vi "read_csv.vi"(7 "Read":bool, 11 "Read File:":path) -> (1 "Header":string[][](array[string]), 2 "# Header Lines":i32, 3 "File Data":T1)   [LabVIEW 2019]
uses:
  <vilib>/Analysis/Matrix/Datatypes/RealMatrix.ctl
  <vilib>/Utility/file.llb/Read Delimited Spreadsheet (DBL).vi
  <vilib>/Utility/file.llb/Read Delimited Spreadsheet (string).vi
  <vilib>/Analysis/Matrix/Numeric/Conversions/Array To Matrix - RA2.vi
  <vilib>/Analysis/Matrix/NI_Matrix.lvlib
panel:
  out "Head Row?":bool
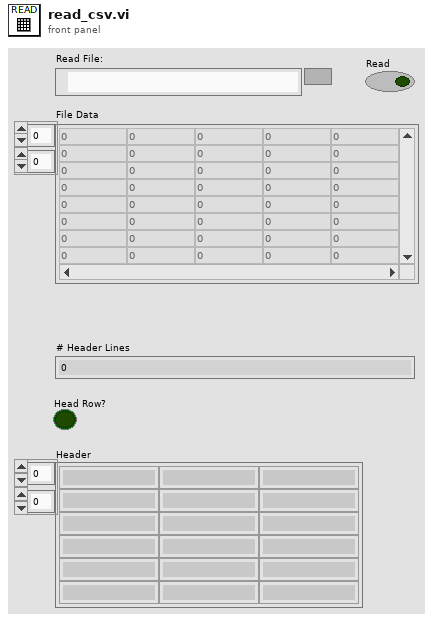
[diagram p1: front panel]
types:
  T1 = typedef "NI_Matrix.lvlib/RealMatrix.ctl" = dbl[][]
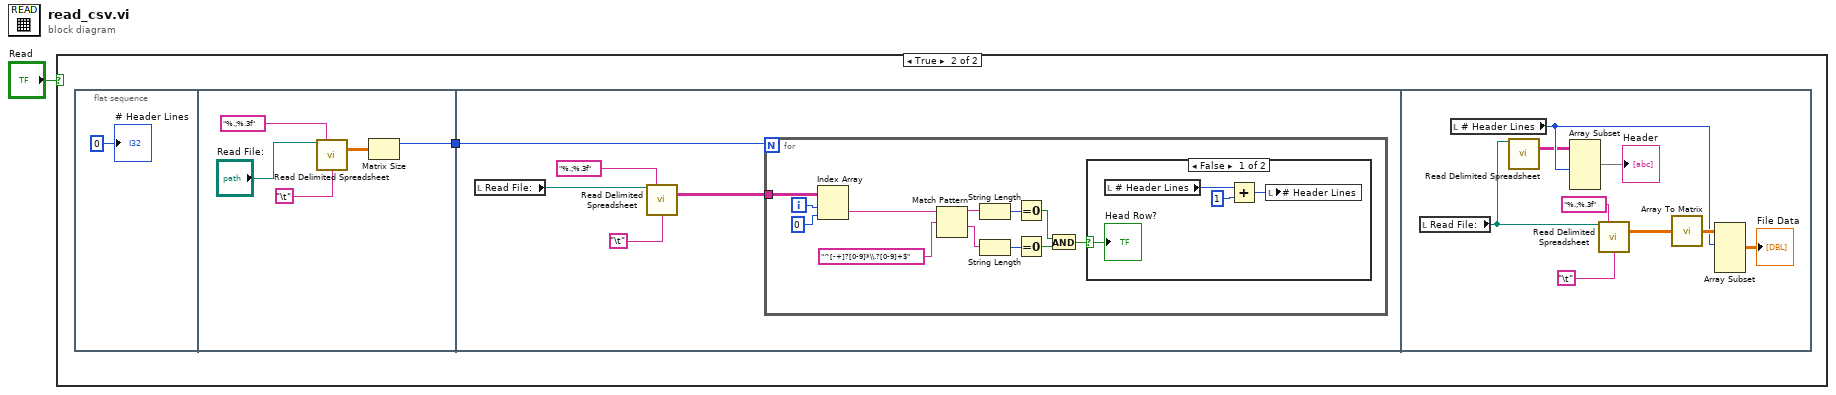
[diagram p0: block diagram]
diagram:
  n1 = case shown="True" "Read" {
    frame False {
    }
    frame True {
      n2 = flat-sequence {
        tunnel: [w4] -> w2
        tunnel: w2 -> [w9]
        frame #0 {
          "# Header Lines" <- 0 ("Header Lines")
        }
        frame #1 {
          n3 = call-poly <vilib>:"Read Delimited Spreadsheet.vi"("file path (dialog if empty)"="Read File:", "format (%.3f)"="%.;%.3f", "delimiter (\\t)"="\t") -> ("all rows"=w8:dbl[][])  [unwired: 7 in, 5 out]
          n4 = Matrix Size(0:w8) -> (1:w4:i32)  [unwired: 1 out]
        }
        frame #2 {
          n5 = local read "Read File:"() -> (w10:path)
          n6 = call-poly <vilib>:"Read Delimited Spreadsheet.vi"("file path (dialog if empty)"=w10, "format (%s)"="%.;%.3f", "delimiter (\\t)"="\t") -> ("all rows"=w13:string[][])  [unwired: 7 in, 5 out]
          n7 = for {
            N: w9 -> [_]
            tunnel: w13 -> [w25]
            i -> [w15]
            n8 = Index Array(array=w25, index (row)=w15, index (col)=0 ("disabled index (col)")) -> (element=w18:string)
            n9 = Match Pattern(string=w18, regular expression="^[-+]?[0-9]*\\.?[0-9]+$") -> (before substring=w19:string, after substring=w20:string)  [unwired: 1 in, 2 out]
            n10 = String Length(string=w19) -> (length=w24:i32)
            n11 = String Length(string=w20) -> (length=w23:i32)
            n12 = Equal To 0?(x=w24) -> (x = 0?=w21:bool)
            n13 = Equal To 0?(x=w23) -> (x = 0?=w22:bool)
            n14 = And(x=w21, y=w22) -> (x .and. y?=w16:bool)
            n15 = case shown="False" w16 {
              selector: w16 -> [w26 _]
              frame False {
                n16 = local read "# Header Lines"() -> (w27:i32)
                n17 = Add(x=w27, y=1) -> (x+y=w29:i32)
                n18 = local write "# Header Lines"(w29) -> ()
                "Head Row?" <- w26
              }
              frame True {
              }
            }
          }
        }
        frame #3 {
          n19 = local read "Read File:"() -> (w33:path)
          n20 = local read "# Header Lines"() -> (w32:i32)
          n21 = call-poly <vilib>:"Read Delimited Spreadsheet.vi"("file path (dialog if empty)"=w33) -> ("all rows"=w31:string[][])  [unwired: 9 in, 5 out]
          n22 = Array Subset(array=w31, length (row)=w32) -> (→"Header":string[][])  [unwired: 3 in]
          n23 = call-poly <vilib>:"Read Delimited Spreadsheet.vi"("file path (dialog if empty)"=w33, "format (%.3f)"="%.;%.3f", "delimiter (\\t)"="\t") -> ("all rows"=w38:dbl[][])  [unwired: 7 in, 5 out]
          n24 = call-poly <vilib>:"Array To Matrix.vi"("Real 2D Array"=w38) -> ("Real Matrix"=w34:T1)
          n25 = Array Subset(array=w34, index (row)=w32) -> (→"File Data":T1)  [unwired: 3 in]
        }
      }
    }
  }
